vi "Performance FGV.vi"(8 "error in (no error)":errorcluster, 11 "Performance Methods":T3) -> (0 "error out":errorcluster, 3 "Performance Data":T1)   [LabVIEW 2017, in "Performance.lvlib"]
uses:
  Performance.lvlib
  Performance Methods.ctl
  Performance Data.ctl
  Dependencies/lv_system_tools/lv_system_tools_100/tools_system CPU Usage Ref.ctl
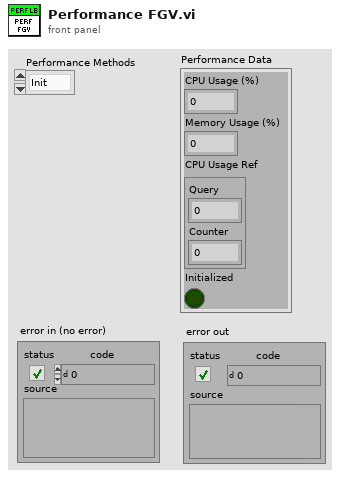
[diagram p1: front panel]
types:
  T1 = typedef "Performance.lvlib/Performance Data.ctl" = cluster{"CPU Usage (%)":dbl, "Memory Usage (%)":dbl, "CPU Usage Ref":T2, "Initialized":bool}
  T2 = typedef "Performance.lvlib/tools_system CPU Usage Ref.ctl" = cluster{"Query":u32, "Counter":u32}
  T3 = typedef "Performance.lvlib/Performance Methods.ctl" = enum16{"Init", "Get Data", "Close"}
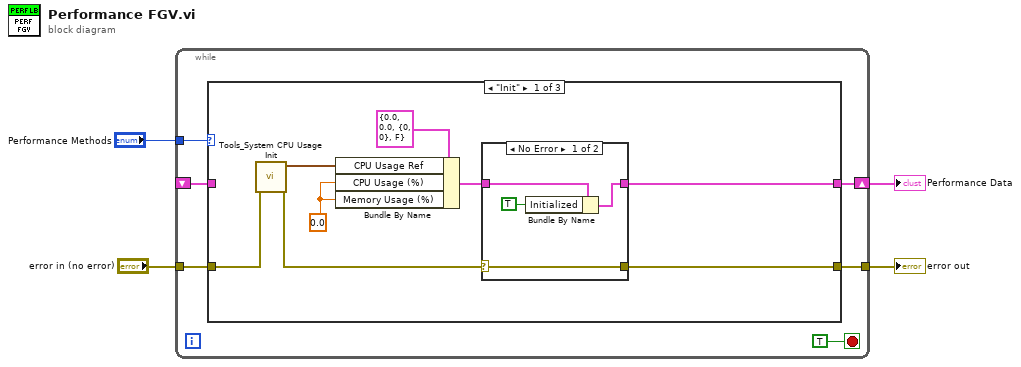
[diagram p0: block diagram]
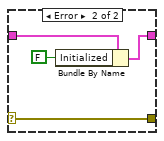
[diagram p2: hidden frame]
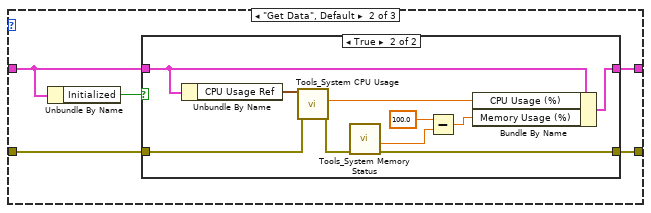
[diagram p3: hidden frame]
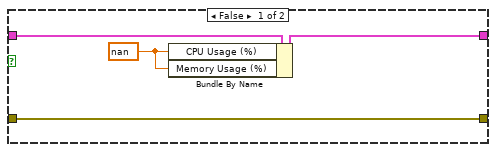
[diagram p4: hidden frame]
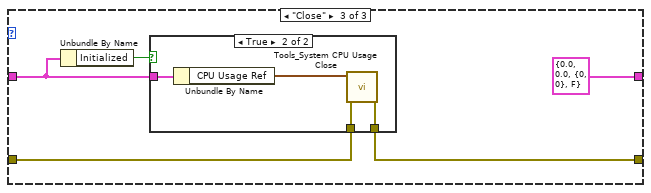
[diagram p5: hidden frame]
diagram:
  n1 = while {
    tunnel: "Performance Methods" -> [w9]
    tunnel: "error in (no error)" -> [w8]
    tunnel: [w7] -> w2
    shift-right: [w6] -> w1
    shift-left: _ -> [w5]
    stop <- TRUE stop-if-true
    n2 = case shown="\"Init\"" w9 {
      tunnel: w8 -> [w18 w30 w50]
      tunnel: [w13 w29 w49] -> w7
      tunnel: [w11 w31 T1 {"CPU Usage (%)"=0.0, "Memory Usage (%)"=0.0, "CPU Usage Ref"={"Query"=0, "Counter"=0}, "Initialized"=FALSE} ("Performance Data")] -> w6
      tunnel: w5 -> [_ w28 w47]
      frame "Init" {
        w16 = 0.0 ("CPU Usage")
        n3 = call "Tools_System CPU Usage Init.vi"("error in (no error)"=w18) -> ("error out"=w14:errorcluster, "CPU Usage Ref"=w15:T2)  [unwired: 9 in]
        n4 = Bundle By Name(cluster=T1 {"CPU Usage (%)"=0.0, "Memory Usage (%)"=0.0, "CPU Usage Ref"={"Query"=0, "Counter"=0}, "Initialized"=FALSE} ("Performance Data"), "CPU Usage Ref"=w15, "CPU Usage (%)"=w16, "Memory Usage (%)"=w16) -> (w12:T1)
        n5 = case shown="No Error" w14 {
          selector: w14 -> [w22 w26]
          tunnel: [w22 w26] -> w13
          tunnel: w12 -> [w21 w25]
          tunnel: [w20 w24] -> w11
          frame No Error {
            n6 = Bundle By Name(cluster=w21, "Initialized"=TRUE) -> (w20:T1)
          }
          frame Error {
            n7 = Bundle By Name(cluster=w25, "Initialized"=FALSE) -> (w24:T1)
          }
        }
      }
      frame "Get Data", Default {
        n8 = Unbundle By Name(w28) -> ("Initialized"=w27:bool)
        n9 = case shown="True" w27 {
          tunnel: [w33 w45] -> w31
          tunnel: w30 -> [w34 w44]
          tunnel: w28 -> [w35 w43]
          tunnel: [w34 w40] -> w29
          frame False {
            w32 = nan ("CPU Usage")
            n10 = Bundle By Name(cluster=w35, "CPU Usage (%)"=w32, "Memory Usage (%)"=w32) -> (w33:T1)
          }
          frame True {
            n11 = Unbundle By Name(w43) -> ("CPU Usage Ref"=w42:T2)
            n12 = call "Tools_System CPU Usage.vi"("error in"=w44, "CPU Usage Ref"=w42) -> ("error out"=w41:errorcluster, "CPU Usage (%)"=w39:dbl)  [unwired: 7 in, 1 out]
            n13 = call "Tools_System Memory Status.vi"("error in (no error)"=w41) -> ("error out"=w40:errorcluster, "Free memory (%)"=w38:dbl)  [unwired: 7 in, 2 out]
            n14 = Subtract(x=100.0, y=w38) -> (x-y=w36:dbl)
            n15 = Bundle By Name(cluster=w43, "CPU Usage (%)"=w39, "Memory Usage (%)"=w36) -> (w45:T1)
          }
        }
      }
      frame "Close" {
        n16 = Unbundle By Name(w47) -> ("Initialized"=w46:bool)
        n17 = case shown="True" w46 {
          tunnel: w50 -> [w51 w55]
          tunnel: [w51 w54] -> w49
          tunnel: w47 -> [_ w53]
          frame False {
          }
          frame True {
            n18 = Unbundle By Name(w53) -> ("CPU Usage Ref"=w52:T2)
            n19 = call "Tools_System CPU Usage Close.vi"("error in"=w55, "CPU Usage Ref"=w52) -> ("error out"=w54:errorcluster)  [unwired: 9 in]
          }
        }
      }
    }
  }
  "error out" <- w2
  "Performance Data" <- w1
